vi "Update monochromator API.vi"(7 "Monochromator":T1={"Type"=enum."PTI", "Wavelength (nm)"=600.0, "Wavelength (nm)"="600 nm", "Grating, gr/mm"=2, "Grating mode"=enum."unknown", "Spectrum mode"={"Spectrum mode?"=FALSE, "Start wavelength (nm)"=0.0, "End wavelength (nm)"=0.0, "Wavelength step (nm)"=0.0, "Wavelength array"=[], "array index"=0}, "VISA"={"delay before read (ms)"=50, "Mono 1"={"Enable Termination Char (T)"=FALSE, "timeout (msec)"=1000, "Resource name"="COM1", "baud rate"=9600, "data bits"=8, "parity"=0, "stop bits"=10, "flow control"=0}, "Mono 2"={"Enable Termination Char (T)"=FALSE, "timeout (msec)"=1000, "Resource name"="COM1", "baud rate"=9600, "data bits"=8, "parity"=0, "stop bits"=10, "flow control"=0}}} {"VISA"."Mono 2"."flow control" items=["None"=0, "XON/XOFF"=1, "RTS/CTS"=2, "DTR/DSR"=4]; "VISA"."Mono 2"."stop bits" items=["None"=0, "XON/XOFF"=1, "RTS/CTS"=2, "DTR/DSR"=4]; "VISA"."Mono 2"."parity" items=["1.0"=10, "1.5"=15, "2.0"=20]; "VISA"."Mono 1"."flow control" items=["None"=0, "XON/XOFF"=1, "RTS/CTS"=2, "DTR/DSR"=4]; "VISA"."Mono 1"."stop bits" items=["None"=0, "XON/XOFF"=1, "RTS/CTS"=2, "DTR/DSR"=4]; "VISA"."Mono 1"."parity" items=["1.0"=10, "1.5"=15, "2.0"=20]; "Grating, gr/mm" items=["2400", "1800", "1200", "600", "300", "150"]}, 8 "Error In":errorcluster) -> (0 "Error Out":errorcluster)   [LabVIEW 2017]
uses:
  Monochromator/Controls/Params.ctl
  Monochromator/Controls/Grating.ctl
  Monochromator/Controls/VISA parameters.ctl
  Controls/Command Data [cluster].ctl
  Controls/Commands [enum].ctl
  System Control/System Control Module.lvlib
  UI.lvlib
  Serial comms/Serial comms.lvlib
  Monochromator/Monochromator.lvlib
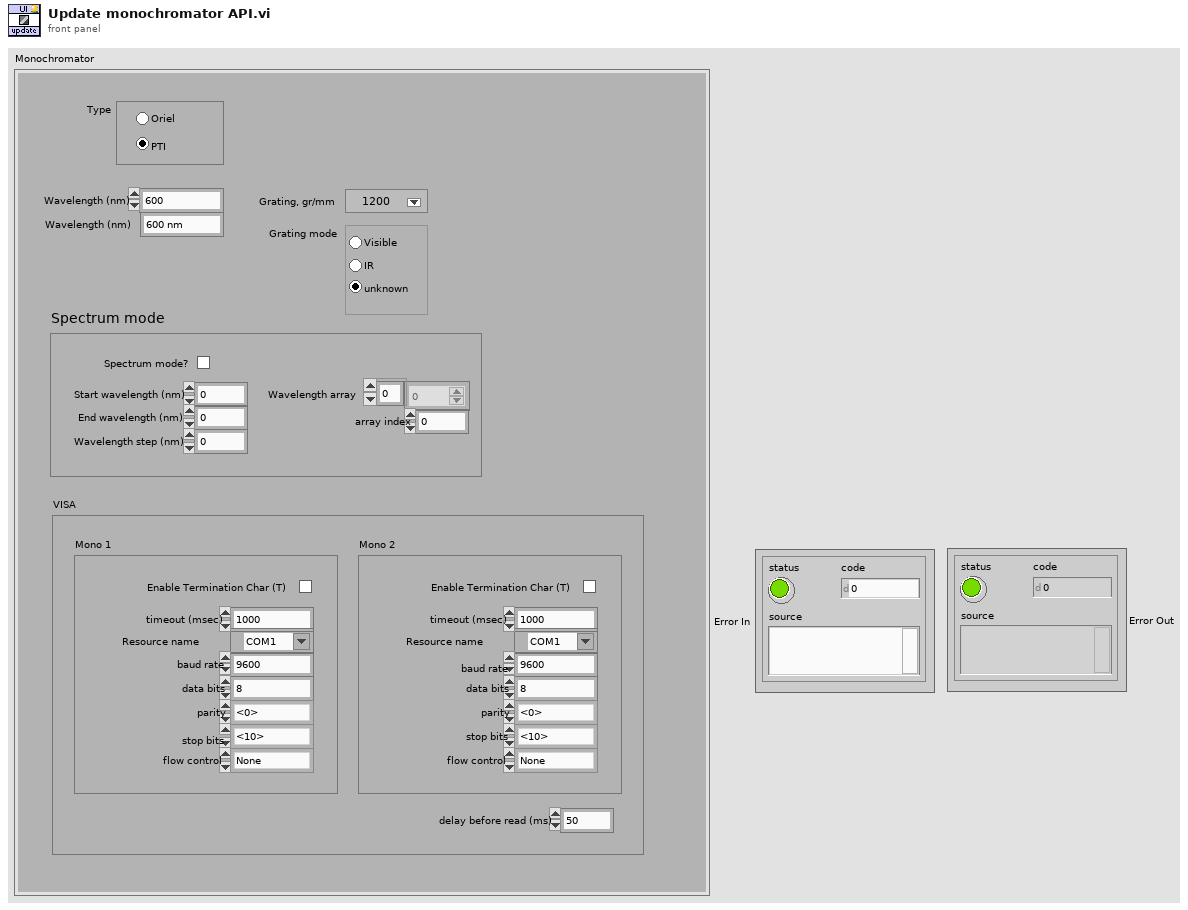
[diagram p1: front panel]
types:
  T1 = typedef "Monochromator.lvlib/Params.ctl" = cluster{"Type":enum32{"Oriel", "PTI"}, "Wavelength (nm)":dbl, "Wavelength (nm)":string, "Grating, gr/mm":u16, "Grating mode":T2, "Spectrum mode":cluster{"Spectrum mode?":bool, "Start wavelength (nm)":dbl, "End wavelength (nm)":dbl, "Wavelength step (nm)":dbl, "Wavelength array":dbl[], "array index":u32}, "VISA":cluster{"delay before read (ms)":u32, "Mono 1":T3, "Mono 2":T3}}
  T2 = typedef "Monochromator.lvlib/Grating.ctl" = enum32{"unknown", "Visible", "IR"}
  T3 = typedef "Serial comms.lvlib/VISA parameters.ctl" = cluster{"Enable Termination Char (T)":bool, "timeout (msec)":u32, "Resource name":refnum<visa-resource-name>, "baud rate":u32, "data bits":u16, "parity":u16, "stop bits":u16, "flow control":u16}
  T4 = typedef "UI.lvlib/Command Data [cluster].ctl" = cluster{"Command":T5, "Data":variant}
  T5 = typedef "UI.lvlib/Commands [enum].ctl" = enum16{"Start", "Update", "Stop"}
  T6 = typedef "System Control Module.lvlib/User Event Refs [cluster].ctl" = cluster{"Exit":refnum<user-event>, "Controller":refnum<user-event>, "System Error":refnum<user-event>, "UI":refnum<user-event>, "Example Module":refnum<user-event>, "Shutter":refnum<user-event>, "Monochromator":refnum<user-event>, "DAQ":refnum<user-event>, "Example Module 2":refnum<user-event>}
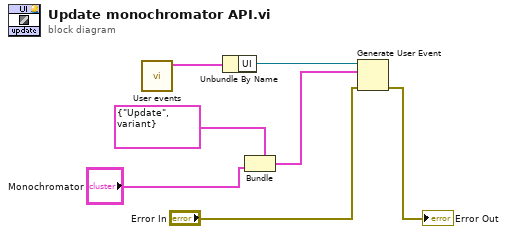
[diagram p0: block diagram]
diagram:
  n1 = call "User events.vi"() -> ("Messages"=w7:T6)  [unwired: 10 in, 1 out]
  n2 = Unbundle By Name(w7) -> ("UI"=w6:refnum<user-event>)
  n3 = Bundle(cluster=T4 {"Command"=enum."Update", "Data"=variant} ("event data"), "Data"="Monochromator") -> (w2:T4)  [unwired: 1 in]
  n4 = Generate User Event(user event=w6, event data cluster=w2, error in="Error In") -> (error out=→"Error Out":errorcluster)  [unwired: 1 in, 1 out]
